vi "setListBox_width_length.vi"(8 "error in (no error)":errorcluster, 10 "Lengths":i32[](array[numeric])=[4, 23, 8, 7, 11, 11, 6, 5, 9, 3, 3, 4, 6, 7, 9, 7, 7], 11 "MCListbox Refnum":refnum<vi>) -> (0 "error out":errorcluster)   [LabVIEW 2019]
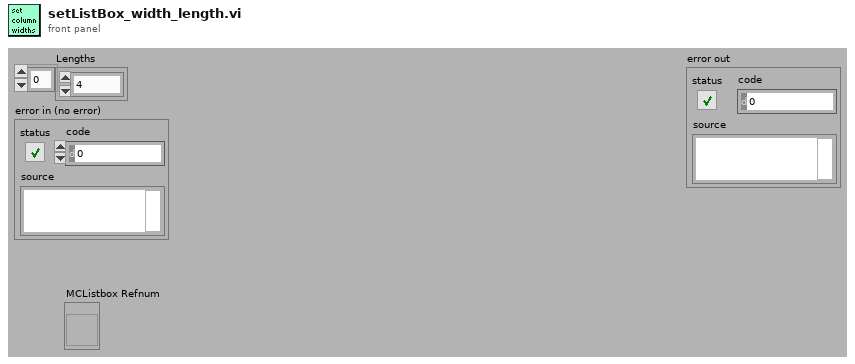
[diagram p1: front panel]
types:
  T1 = cluster{"Font Name:":string, "Size":i16, "Strikeout?":bool, "Italic?":bool, "Underline?":bool, "Outline?":bool, "Shadow?":bool, "Bold?":bool}
  T2 = enum16{"User-specified Font", "Application Font", "System Font", "Dialog Font"}
  T3 = typedef "LVFontTypeDef.ctl" = cluster{"Font Name":string, "Size":u16, "Bold":bool, "Italic":bool, "Underline":bool, "Strikeout":bool, "Color":u32}
  T4 = cluster{"left":i16, "top":i16, "right":i16, "bottom":i16}
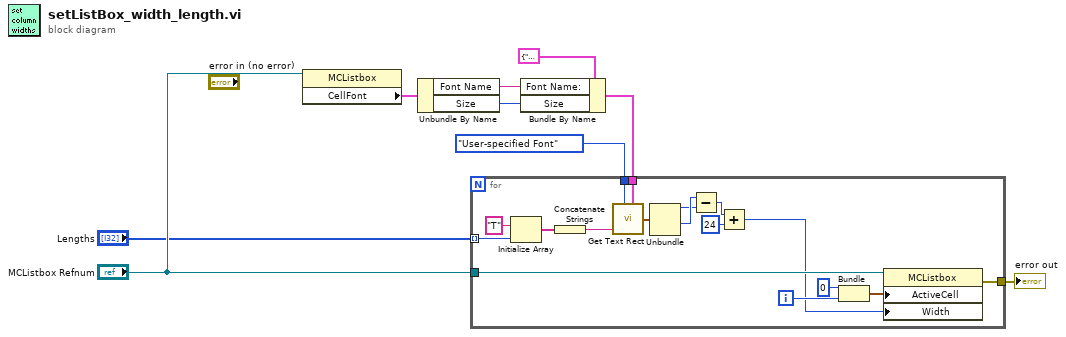
[diagram p0: block diagram]
diagram:
  n1 = property on="Property Node" class="MCListbox"(reference="MCListbox Refnum") -> ("CellFont"=w6:T3)  [unwired: 1 in, 2 out]
  n2 = Unbundle By Name(w6) -> ("Font Name"=w4:string, "Size"=w3:u16)
  n3 = Bundle By Name(cluster=T1 {"Font Name:"="", "Size"=0, "Strikeout?"=FALSE, "Italic?"=FALSE, "Underline?"=FALSE, "Outline?"=FALSE, "Shadow?"=FALSE, "Bold?"=FALSE} ("[user-specified font]"), "Font Name:"=w4, "Size"=w3) -> (w5:T1)
  n4 = for {
    tunnel: "MCListbox Refnum" -> [w23]
    tunnel: [w22] -> w1
    tunnel: T2."User-specified Font" ("desired font(Application)") -> [w21]
    tunnel: w5 -> [w20]
    tunnel: "Lengths" -> [w19] mode=indexing
    i -> [w24]
    n5 = Initialize Array("T" ("Font Name"), w19) -> (w17:string[])
    n6 = Concatenate Strings(w17) -> (w11:string)
    n7 = call <vilib>:"Get Text Rect.vi"("desired font(Application)"=w21, "text"=w11, "[user-specified font]"=w20) -> ("rect"=w16:T4)  [unwired: 6 in]
    n8 = Unbundle(w16) -> ("left"=w14:i16, "right"=w15:i16)  [unwired: 2 out]
    n9 = Subtract(x=w15, y=w14) -> (x-y=w13:i16)
    n10 = Add(x=w13, y=i16 24) -> (x+y=w10:i16)
    n11 = Bundle(0, w24) -> (w26:cluster{i32, i32})  [unwired: 1 in]
    n12 = property on="Property Node" class="MCListbox"(reference=w23, "ActiveCell"=w26, "Width"=w10) -> (error out=w22:errorcluster)  [unwired: 1 in, 1 out]
  }
  "error out" <- w1
